vi "WriteV_60Series12.vi"() -> ()   [LabVIEW 2019]
panel:
  out "read buffer":string
  in  "stop":bool
  out "Measured Voltage 1":sgl
  in  "Supply Voltage":dbl
  out "error out":errorcluster
  in  "error in (no error)":errorcluster
  in  "VISA resource name":refnum<visa-resource-name>
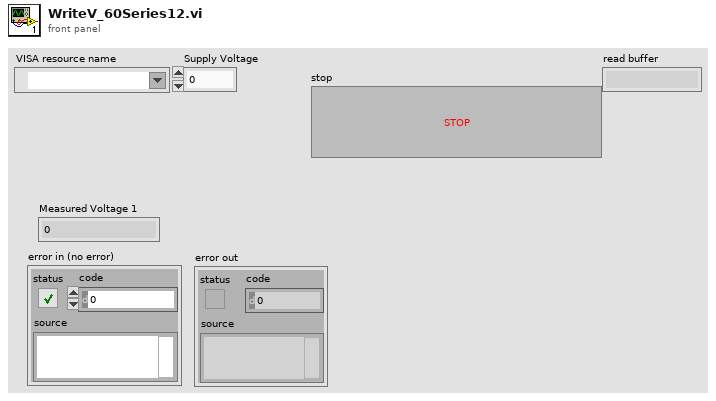
[diagram p1: front panel]
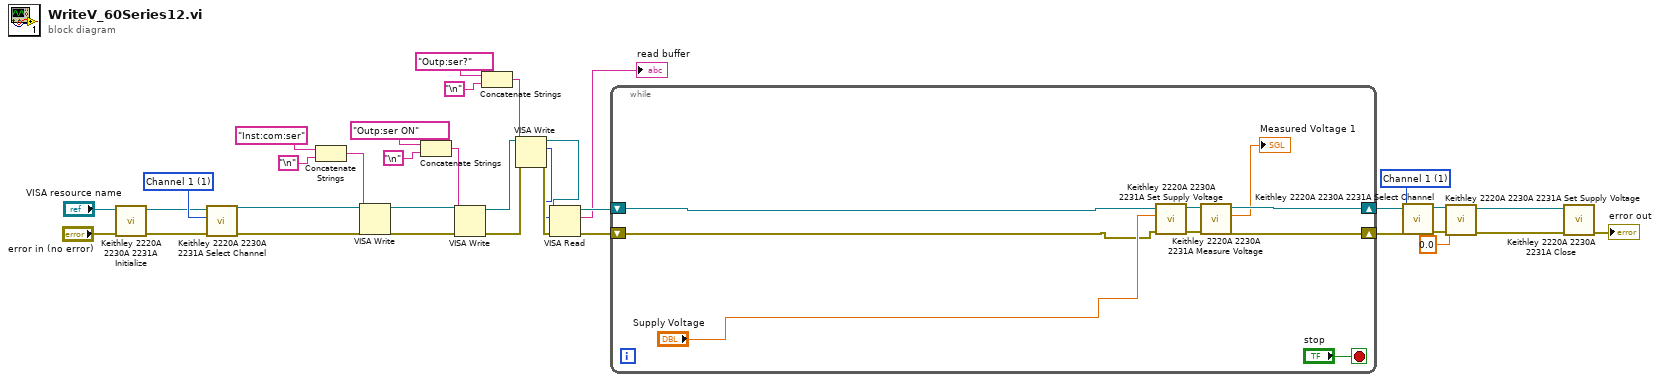
[diagram p0: block diagram]
diagram:
  w5 = u16 1 items=["N/A", "Channel 1", "Channel 2", "Channel 3"] ("Channel Control")
  w30 = u16 1 items=["N/A", "Channel 1", "Channel 2", "Channel 3"] ("Channel Control")
  n1 = call "Keithley 2220A 2230A 2231A Initialize.vi"("error in (no error)"="error in (no error)", "VISA resource name"="VISA resource name") -> ("error out"=w3:errorcluster, "VISA resource name out"=w4:refnum<visa-resource-name>)  [unwired: 7 in, 1 out]
  n2 = call "Keithley 2220A 2230A 2231A Select Channel.vi"("error in (no error)"=w3, "Channel Control"=w5, "VISA resource name"=w4) -> ("error out"=w2:errorcluster, "VISA resource name out"=w1:refnum<visa-resource-name>)  [unwired: 7 in]
  n3 = Concatenate Strings("Inst:com:ser" ("string"), "\n") -> (w25:string)
  n4 = VISA Write(VISA resource name=w1, write buffer=w25, error in (no error)=w2) -> (VISA resource name out=w19:refnum<visa-resource-name>, error out=w20:errorcluster)  [unwired: 1 out]
  n5 = Concatenate Strings("Outp:ser ON" ("string"), "\n") -> (w22:string)
  n6 = VISA Write(VISA resource name=w19, write buffer=w22, error in (no error)=w20) -> (VISA resource name out=w10:refnum<visa-resource-name>, error out=w9:errorcluster)  [unwired: 1 out]
  n7 = Concatenate Strings("Outp:ser?" ("string"), "\n") -> (w12:string)
  n8 = VISA Write(VISA resource name=w10, write buffer=w12, error in (no error)=w9) -> (VISA resource name out=w6:refnum<visa-resource-name>, return count=w7:u32, error out=w8:errorcluster)
  n9 = VISA Read(VISA resource name=w6, byte count=w7, error in (no error)=w8) -> (VISA resource name out=w16:refnum<visa-resource-name>, read buffer=→"read buffer":string, error out=w15:errorcluster)  [unwired: 1 out]
  n10 = while {
    shift-right: [w44] -> w31
    shift-left: w15 -> [w36]
    shift-right: [w43] -> w32
    shift-left: w16 -> [w37]
    stop <- "stop" stop-if-true
    n11 = call "Keithley 2220A 2230A 2231A Set Supply Voltage.vi"("error in (no error)"=w36, "Supply Voltage"="Supply Voltage", "VISA resource name"=w37) -> ("error out"=w39:errorcluster, "VISA resource name out"=w38:refnum<visa-resource-name>)  [unwired: 7 in]
    n12 = call "Keithley 2220A 2230A 2231A Measure Voltage.vi"("error in (no error)"=w39, "VISA resource name"=w38) -> ("error out"=w44:errorcluster, "Measured Voltage"=→"Measured Voltage 1":sgl, "VISA resource name out"=w43:refnum<visa-resource-name>)  [unwired: 7 in]
  }
  n13 = call "Keithley 2220A 2230A 2231A Select Channel.vi"("error in (no error)"=w31, "Channel Control"=w30, "VISA resource name"=w32) -> ("error out"=w29:errorcluster, "VISA resource name out"=w28:refnum<visa-resource-name>)  [unwired: 7 in]
  n14 = call "Keithley 2220A 2230A 2231A Set Supply Voltage.vi"("error in (no error)"=w29, "Supply Voltage"=0.0, "VISA resource name"=w28) -> ("error out"=w18:errorcluster, "VISA resource name out"=w17:refnum<visa-resource-name>)  [unwired: 7 in]
  n15 = call "Keithley 2220A 2230A 2231A Close.vi"("error in (no error)"=w18, "VISA resource name"=w17) -> ("error out"=→"error out":errorcluster)  [unwired: 9 in]
